vi "Insert LogMeasData in Q.vi"(8 "error in (no error)":errorcluster, 10 "MeasData":T2) -> (0 "error out":errorcluster, 2 "# elements in queue":i32, 3 "orData out":T1)   [LabVIEW 2020]
doc: "Developed by Kevin Thompson\nThompson Engineering, LLC\nkevin@thompsonengineering.net"
uses:
  TD MeasData--cluster.ctl
  TD MeasData QRef.ctl
  GBL DataQ Ref.vi
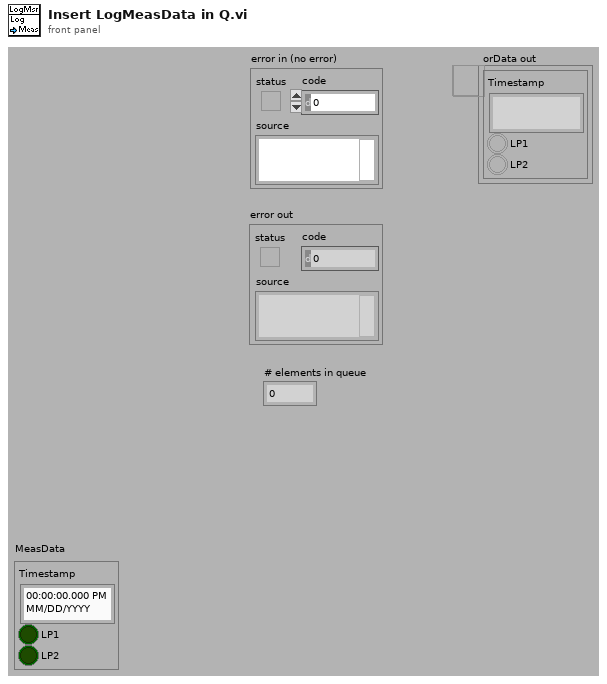
[diagram p1: front panel]
types:
  T1 = typedef "TD MeasData QRef.ctl" = refnum<queue>
  T2 = typedef "TD MeasData--cluster.ctl" = cluster{"Timestamp":timestamp, "LP1":bool, "LP2":bool}
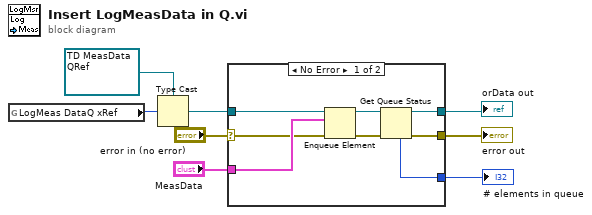
[diagram p0: block diagram]
diagram:
  n1 = global read "GBL DataQ Ref.vi" "LogMeas DataQ xRef"() -> (w2:u32)
  n2 = Type Cast(type=T1 refnum ("orData in"), x=w2) -> (*(type *) &x=w5:T1)
  n3 = case shown="No Error" "error in (no error)" {
    selector: "error in (no error)" -> [w13 w17]
    tunnel: w5 -> [w15 w18]
    tunnel: [w10 w17] -> w8
    tunnel: [w12 w18] -> w6
    tunnel: "MeasData" -> [w14 _]
    tunnel: [w9 _] -> w1
    frame No Error {
      n4 = Enqueue Element(queue=w15, element=w14, error in (no error)=w13) -> (queue out=w16:T1, error out=w11:errorcluster)  [unwired: 1 in, 1 out]
      n5 = Get Queue Status(queue=w16, error in (no error)=w11) -> (queue out=w12:T1, error out=w10:errorcluster, # elements in queue=w9:i32)  [unwired: 1 in, 5 out]
    }
    frame Error {
    }
  }
  "error out" <- w8
  "orData out" <- w6
  "# elements in queue" <- w1
